vi "Convert Image pixel_v2.vi"(7 "serial channel display parameters":T1[](array[typedef]) {"RAW parameters"."bayer parameters"."blue gain" format="%_4g"; "RAW parameters"."bayer parameters"."green gain" format="%_4g"; "RAW parameters"."bayer parameters"."red gain" format="%_4g"; "RAW parameters"."bayer parameters"."algorithm" items=["Bilinear", "VNG"]; "RAW parameters"."bayer parameters"."pattern" items=["GB", "GR", "BG", "RG"]}, 8 "error in":errorcluster, 10 "image metadata":T4, 11 "Refnum in":T2) -> (0 "error out":errorcluster, 3 "Image Pixels (U32)":u32[](array[numeric]))   [LabVIEW 2025, in "Automotive Vision.lvclass"]
doc: "Convert an image to U32 array corresponds to image type."
uses:
  Automotive Vision.lvclass
  Automotive Vision.lvclass/Automotive Vision.ctl
  deps/NI148X/Getting Started/Host/Common/Types/RAW Interpretation for Display.ctl
  deps/NI148X/Getting Started/Host/Common/GettingStarted_Common_148X_Host.lvlib
  <instrlib>/FlexRIO/CSI-2/v2/Common/Types/LLP Data Type.ctl
  <instrlib>/FlexRIO/CSI-2/v2/Common/NI CSI-2 API Common v2.lvlib
  deps/NI148X/Getting Started/FPGA/Common/Types/Image Metadata.ctl
  deps/NI148X/Getting Started/FPGA/Common/GettingStarted_Common_148X_FPGA.lvlib
  <vilib>/vision/Image Controls.llb/IMAQ Image.ctl
  deps/NI148X/Getting Started/Host/Common/Types/Serial Channel Display Parameters.ctl
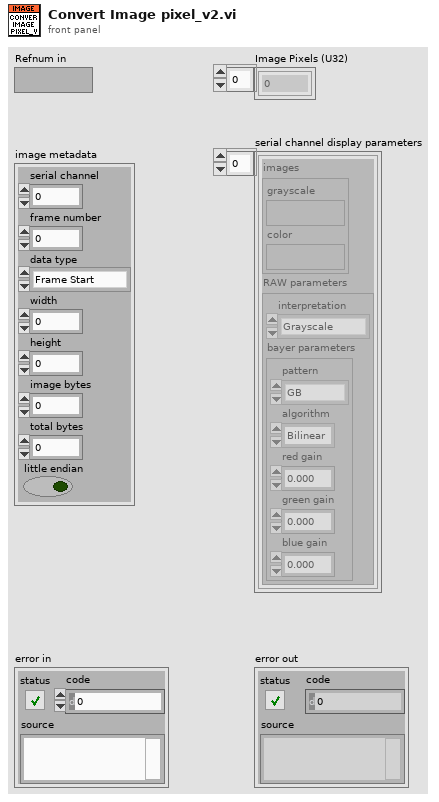
[diagram p1: front panel]
types:
  T1 = typedef "GettingStarted_Common_148X_Host.lvlib/Serial Channel Display Parameters.ctl" = cluster{"images":cluster{"grayscale":T2, "color":T2}, "RAW parameters":cluster{"interpretation":T3, "bayer parameters":cluster{"pattern":i32, "algorithm":i32, "red gain":dbl, "green gain":dbl, "blue gain":dbl}}}
  T2 = typedef "IMAQ Image.ctl" = refnum<image>
  T3 = typedef "GettingStarted_Common_148X_Host.lvlib/RAW Interpretation for Display.ctl" = enum16{"Grayscale", "Bayer", "RGB", "YUV422", "YUV420", "Legacy YUV420"}
  T4 = typedef "GettingStarted_Common_148X_FPGA.lvlib/Image Metadata.ctl" = cluster{"serial channel":fxp<+,3,3>, "frame number":u16, "data type":T5, "width":u16, "height":u16, "image bytes":u32, "total bytes":u32, "little endian":bool}
  T5 = typedef "NI CSI-2 API Common v2.lvlib/LLP Data Type.ctl" = enum8{"Frame Start", "Frame End", "Line Start", "Line End", "End of Transmission", "Reserved 0", "Reserved 1", "Reserved 2", "Generic Short Packet 1", "Generic Short Packet 2", "Generic Short Packet 3", "Generic Short Packet 4", "Generic Short Packet 5", "Generic Short Packet 6", "Generic Short Packet 7", "Generic Short Packet 8", "Null", "Blanking Data", "Embedded 8-bit non Image Data", "Generic Long Packet 1", "Generic Long Packet 2", "Generic Long Packet 3", "Generic Long Packet 4", "Reserved 3", "YUV420 8-bit", "YUV420 10-bit", "Legacy YUV420 8-bit", "Reserved 4", "YUV420 8-bit Chroma Shifted", "YUV420 10-bit Chroma Shifted", "YUV422 8-bit", "YUV422 10-bit", "RGB444", "RGB555", "RGB565", "RGB666", "RGB888", "Reserved 5", "Reserved 6", "RAW 24", "RAW 6", "RAW 7", "RAW 8", "RAW 10", "RAW 12", "RAW 14", "RAW 16", "RAW 20", "User Defined 8-bit Data 1", "User Defined 8-bit Data 2", "User Defined 8-bit Data 3", "User Defined 8-bit Data 4", "User Defined 8-bit Data 5", "User Defined 8-bit Data 6", "User Defined 8-bit Data 7", "User Defined 8-bit Data 8", "USL Command", "Reserved 7", "Reserved 8", "Reserved 9", "Reserved 10", "Reserved 11", "Reserved 12", "LRTE EPD Spacer"}
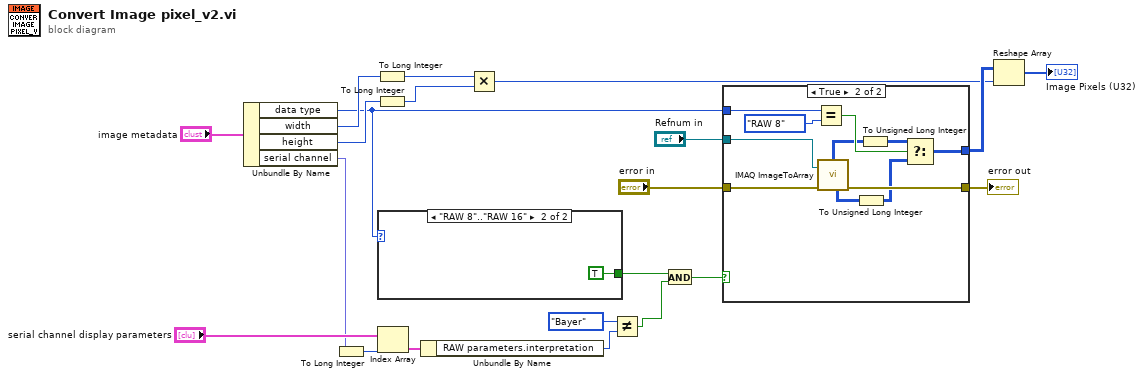
[diagram p0: block diagram]
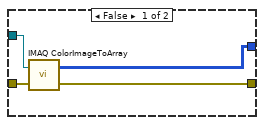
[diagram p3: hidden frame]
diagram:
  n1 = Unbundle By Name("image metadata") -> ("data type"=w6:T5, "width"=w10:u16, "height"=w11:u16, "serial channel"=w1:fxp<+,3,3>)
  n2 = To Long Integer(number=w1) -> (32bit integer=w2:i32)
  n3 = To Long Integer(number=w10) -> (32bit integer=w13:i32)
  n4 = To Long Integer(number=w11) -> (32bit integer=w12:i32)
  n5 = case shown="\"RAW 8\"..\"RAW 16\"" w6 {
    tunnel: [_ TRUE] -> w5
    frame "Frame Start", Default {
    }
    frame "RAW 8".."RAW 16" {
    }
  }
  n6 = Index Array(array="serial channel display parameters", index=w2) -> (element=w16:T1)
  n7 = Unbundle By Name(w16) -> ("RAW parameters.interpretation"=w15:T3)
  n8 = Multiply(x=w13, y=w12) -> (x*y=w8:i32)
  n9 = Not Equal?(x=RAW_Interpretation_for_Display."Bayer", y=w15) -> (x != y?=w4:bool)
  n10 = And(x=w5, y=w4) -> (x .and. y?=w3:bool)
  n11 = case shown="True" w3 {
    tunnel: "Refnum in" -> [w26 w36]
    tunnel: [w25 w35] -> w19
    tunnel: "error in" -> [w24 w37]
    tunnel: [w23 w27] -> w9
    tunnel: w6 -> [_ w34]
    frame False {
      n12 = call "IMAQ ColorImageToArray"("Image"=w26, "error in (no error)"=w24) -> ("Image Pixels (U32)"=w23:u32[][], "error out"=w25:errorcluster)  [unwired: 2 in, 1 out]
    }
    frame True {
      n13 = Equal?(x=w34, y=LLP_Data_Type."RAW 8") -> (x = y?=w32:bool)
      n14 = call "IMAQ ImageToArray"("error in (no error)"=w37, "Image"=w36) -> ("Image Pixels (U16)"=w28:u16[][], "error out"=w35:errorcluster, "Image Pixels (U8)"=w31:u8[][])  [unwired: 2 in, 2 out]
      n15 = To Unsigned Long Integer(number=w28) -> (unsigned 32bit integer=w29:u32[][])
      n16 = To Unsigned Long Integer(number=w31) -> (unsigned 32bit integer=w30:u32[][])
      n17 = Select(t=w30, s=w32, f=w29) -> (s? t:f=w27:u32[][])
    }
  }
  "error out" <- w19
  n18 = Reshape Array(w9, w8) -> (→"Image Pixels (U32)":u32[])
